vi "Cycle.vi"(8 "error in (no error)":errorcluster, 11 "PassiveFixation In":refnum<class "PassiveFixation.lvclass">) -> (0 "error out":errorcluster, 3 "PassiveFixation Out":refnum<class "PassiveFixation.lvclass">)   [LabVIEW 2010, in "PassiveFixation.lvclass"]
uses:
  PassiveFixation.lvclass
  PassiveExperiment/PassiveExperiment.lvclass
panel:
  out "XY Graph":cluster{"horizontal":dbl[], "vertical":dbl[]}[](graph)
  in  "Eye Params":dbl[](array[numeric])
  out "Timeouts":T1={"Intertrial"=1000.0, "AcquireFixation"=1000.0, "HoldFixation"=300.0, "DelayPeriod"=1000.0, "ResponsePeriod"=1000.0}
  in  "RewardAmount":dbl=50.0
  in  "FixationRadius":dbl=50.0
  out "ExperimentStats":T2
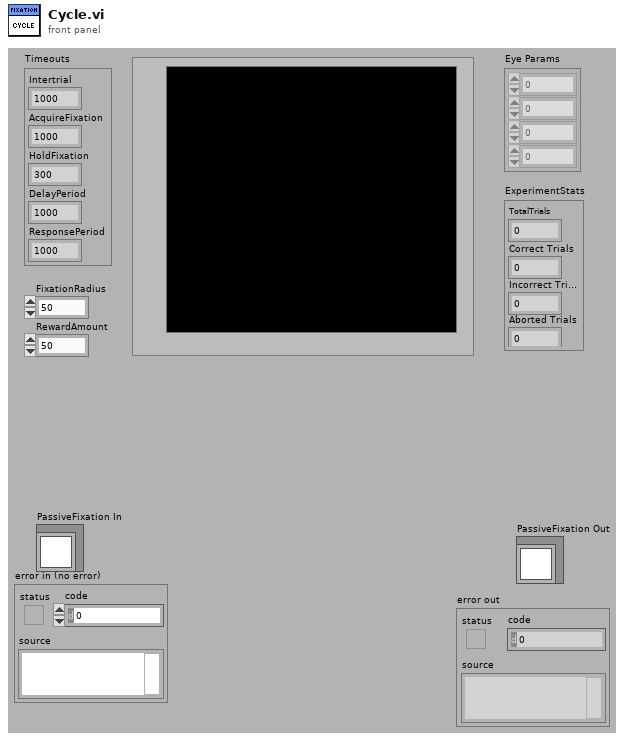
[diagram p1: front panel]
types:
  T1 = cluster{"Intertrial":dbl, "AcquireFixation":dbl, "HoldFixation":dbl, "DelayPeriod":dbl, "ResponsePeriod":dbl}
  T2 = cluster{"TotalTrials":dbl, "Correct Trials":dbl, "Incorrect Trials":dbl, "Aborted Trials":dbl}
  T3 = cluster{"TotalTrials":u32, "Correct Trials":u32, "Incorrect Trials":u32, "Aborted Trials":u32}
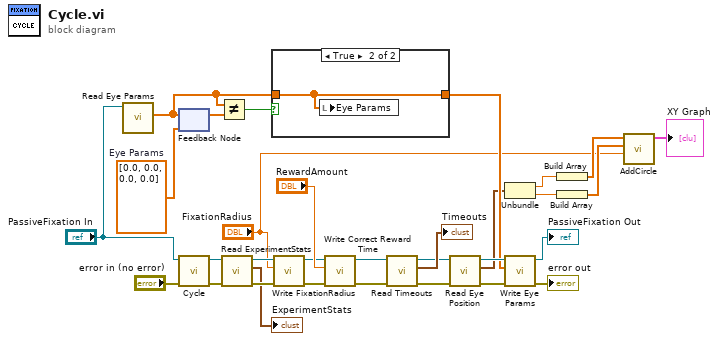
[diagram p0: block diagram]
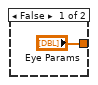
[diagram p2: hidden frame]
diagram:
  w18 = dbl[] [0.0, 0.0, 0.0, 0.0]  # Eye Params
  n1 = call-dynamic "Read Eye Params.vi"("TrialBasedExperiment in"="PassiveFixation In") -> ("Eye Params"=w17:dbl[])  [unwired: 8 in, 2 out]
  n2 = feedback #1(w18) -> (w20:dbl[])
  n3 = feedback-in #1(w17) -> ()
  n4 = call-parent "Cycle.vi"("error in (no error)"="error in (no error)", "PassiveExperiment In"="PassiveFixation In") -> ("error out"=w8:errorcluster, "PassiveExperiment Out"=w7:refnum<class "PassiveFixation.lvclass">)  [unwired: 8 in]
  n5 = Not Equal?(x=w17, y=w20) -> (x != y?=w19:bool)
  n6 = call-dynamic "Read ExperimentStats.vi"("error in (no error)"=w8, "TrialBasedExperiment in"=w7) -> ("error out"=w30:errorcluster, "ExperimentStats"=→"ExperimentStats":T3, "TrialBasedExperiment out"=w31:refnum<class "PassiveFixation.lvclass">)  [unwired: 7 in]
  n7 = case shown="True" w19 {
    tunnel: ["Eye Params" w33] -> w14
    tunnel: w17 -> [_ w33]
    frame False {
    }
    frame True {
      n8 = local write "Eye Params"(w33) -> ()
    }
  }
  n9 = call-dynamic "Write FixationRadius.vi"("error in (no error)"=w30, "FixationRadius"="FixationRadius", "MatlabExperiment in"=w31) -> ("error out"=w27:errorcluster, "MatlabExperiment out"=w28:refnum<class "PassiveFixation.lvclass">)  [unwired: 7 in]
  n10 = call-dynamic "Write Correct Reward Time.vi"("error in (no error)"=w27, "Correct Reward Time"="RewardAmount", "MatlabExperiment in"=w28) -> ("error out"=w25:errorcluster, "MatlabExperiment out"=w26:refnum<class "PassiveFixation.lvclass">)  [unwired: 7 in]
  n11 = call-dynamic "Read Timeouts.vi"("error in (no error)"=w25, "TrialBasedExperiment in"=w26) -> ("error out"=w24:errorcluster, "Timeouts"=→"Timeouts":T1, "TrialBasedExperiment out"=w21:refnum<class "PassiveFixation.lvclass">)  [unwired: 7 in]
  n12 = call-dynamic "Read Eye Position.vi"("error in (no error)"=w24, "TrialBasedExperiment in"=w21) -> ("error out"=w15:errorcluster, "Eye Position"=w11:cluster{"Horizontal":dbl, "Vertical":dbl}, "TrialBasedExperiment out"=w16:refnum<class "PassiveFixation.lvclass">)  [unwired: 7 in]
  n13 = Unbundle(w11) -> ("Horizontal"=w12:dbl, "Vertical"=w13:dbl)
  n14 = call-dynamic "Write Eye Params.vi"("error in (no error)"=w15, "Eye Params"=w14, "TrialBasedExperiment in"=w16) -> ("error out"=→"error out":errorcluster, "TrialBasedExperiment out"=→"PassiveFixation Out":refnum<class "PassiveFixation.lvclass">)  [unwired: 7 in]
  n15 = Build Array(w12) -> (w4:dbl[])
  n16 = Build Array(w13) -> (w3:dbl[])
  n17 = call "AddCircle.vi"("radius"="FixationRadius", "vertical"=w3, "horizontal"=w4) -> ("output"=→"XY Graph":cluster{"horizontal":dbl[], "vertical":dbl[]}[])  [unwired: 8 in]
